vi "test_fit.vi"() -> ()   [LabVIEW 2021]
uses:
  <vilib>/Analysis/Matrix/Datatypes/RealMatrix.ctl
  <vilib>/Analysis/Matrix/NI_Matrix.lvlib
panel:
  out "residue":dbl
  out "covariance":T1 format="%.3f"
  out "number of function calls":i32
  in  "original":dbl[](array[numeric])=[33.0, 0.0, 2.23, 234.0]
  in  "standard deviation":dbl=4.0 format="%0.2f"
  out "coarse estimation":dbl[](array[numeric])
  out "best fit":dbl[](array[numeric])
  in  "termination":cluster{"max iteration":i32, "tolerance":dbl}={"max iteration"=200, "tolerance"=1e-08}
  out "Blah":cluster{"X":dbl[], "f(X;P)":dbl[]}[](graph)
  # "I0\nmu\nw0\nI1"
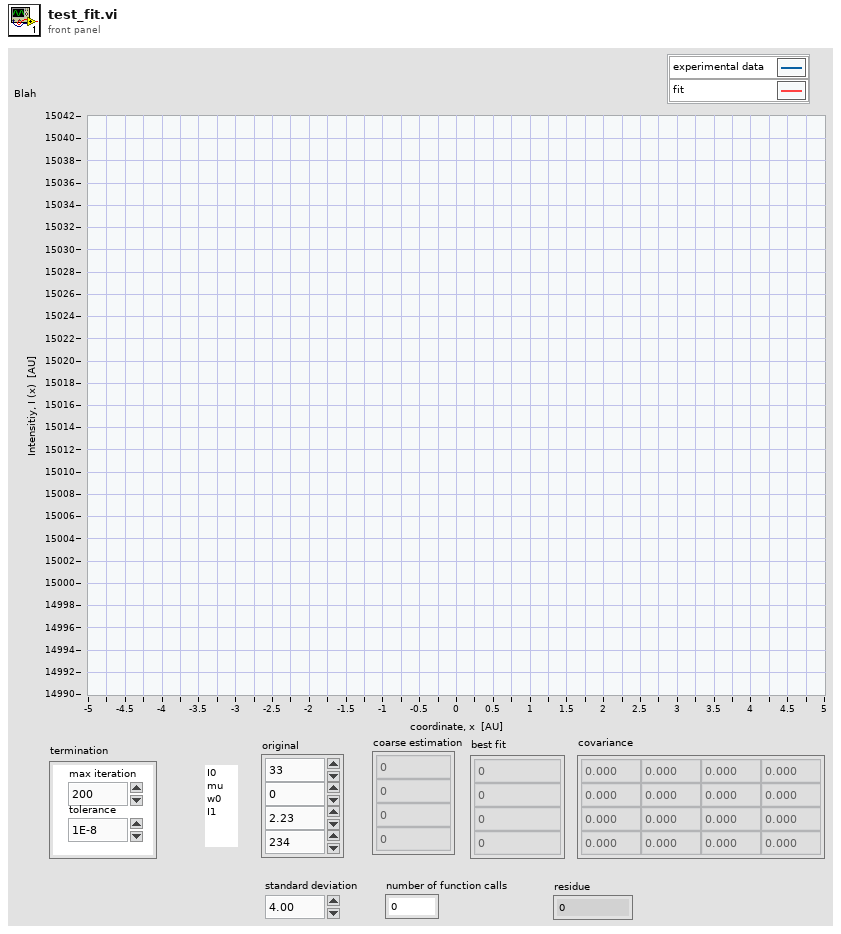
[diagram p1: front panel]
types:
  T1 = typedef "NI_Matrix.lvlib/RealMatrix.ctl" = dbl[][]
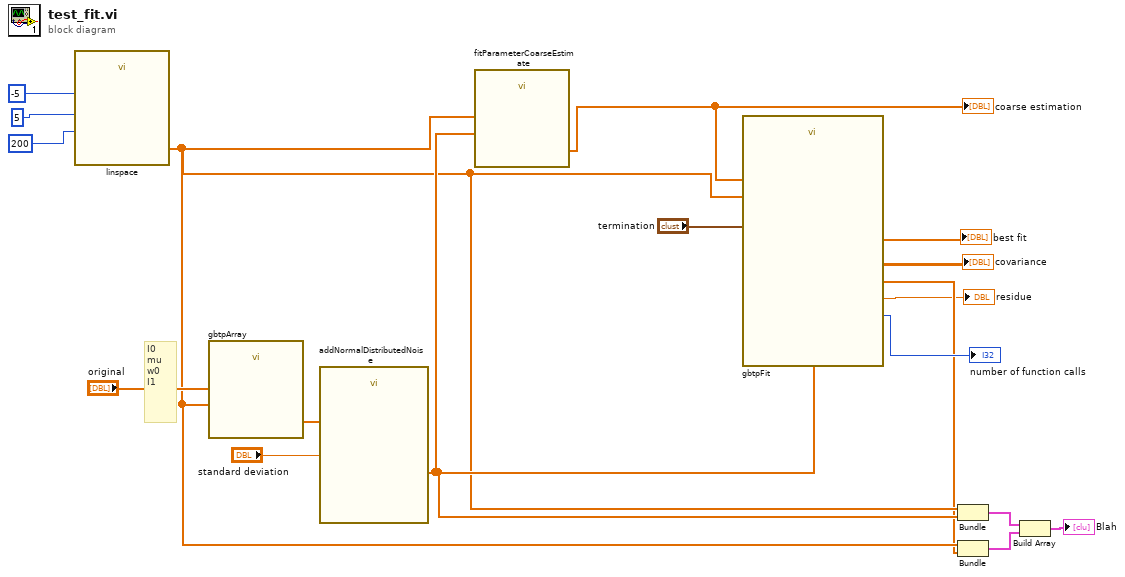
[diagram p0: block diagram]
diagram:
  # "I0\nmu\nw0\nI1"
  n1 = call "linspace.vi"("N"=200 ("step"), "end"=5, "start"=-5) -> ("X"=w9:dbl[])
  n2 = call "gbtpArray.vi"("X"=w9, "P"="original") -> ("f(X;P)"=w8:dbl[])
  n3 = call "addNormalDistributedNoise.vi"("Array"=w8, "standard deviation"="standard deviation") -> ("added Noise Array"=w11:dbl[])  [unwired: 3 in]
  n4 = call "fitParameterCoarseEstimate.vi"("Y"=w11, "X"=w9) -> ("pars"=w12:dbl[])  [unwired: 2 in]
  "coarse estimation" <- w12
  n5 = call "gbtpFit.vi"("Y"=w11, "termination"="termination", "X"=w9, "initial parameters"=w12) -> ("best nonlinear fit"=w2:dbl[], "covariance"=→"covariance":T1, "best fit parameters"=→"best fit":dbl[], "number of function calls"=→"number of function calls":i32, "residue"=→"residue":dbl)  [unwired: 2 in, 1 out]
  n6 = Bundle("X"=w9, "added Noise Array"=w11) -> (w7:cluster{"X":dbl[], "added Noise Array":dbl[]})  [unwired: 1 in]
  n7 = Bundle("X"=w9, "best nonlinear fit"=w2) -> (w6:cluster{"X":dbl[], "best nonlinear fit":dbl[]})  [unwired: 1 in]
  n8 = Build Array(w7, w6) -> (→"Blah":cluster{"X":dbl[], "best nonlinear fit":dbl[]}[])
